vi "dfd_Get Multirate Block Params.vi"(6 "fs in [Hz]":dbl=1.0, 8 "error in (no error)":errorcluster, 9 "type (FLP)":enum16{"FLP", "FXP"}(ring), 11 "multirate filter in":T3={"mMRate_Structure"=enum."CIC", "mMRate_Mode"=0, "mMRate_Factor"=1, "mMRate_FIRParams"={"mMRate_FIR_H"=[], "mMRate_FIR_IsNyquist?"=FALSE, "mMRate_FIR_IsSymmetric?"=FALSE}, "mMRate_CICParams"={"mMRate_CIC_#Stage"=2, "mMRate_CIC_Lag"=1, "mMRate_CIC_Type"=enum."Lowpass"}, "mMRate_Order"=1, "mMRate_Version"="1.0", "mMRate_Comments"="1.0", "mMRate_RationalFactor"={"mMRate_L"=-1, "mMRate_M"=-1}, "mMRate_Fs"=0.0, "mMRate_Quantized?"=FALSE, "mMRate_QFilterGain"=1.0, "mMRate_CoefWl"=16, "mMRate_Scaling"={"mMRate_ScaleByPowerOf2?"=FALSE, "mMRate_ScaleType"=enum."Time Domain 1-Norm"}, "mMRate_InputWl"=0, "mMRate_OutputWl"=0, "mMRate_OutputMode"=enum."Nearest", "mMRate_MultMode"=enum."Truncated", "mMRate_BitPruning"=FALSE, "mMRate_GainWl"=16, "mMRate_OutputFwl"=0, "mMRate_SumIwl"=0, "mMRate_InputIwl "=16, "mMRate_SumWl"=32, "mMRate_CoefIwl"=0} {"mMRate_SumWl" min=1 max=32 step=1; "mMRate_InputIwl" min=1 max=32 step=1; "mMRate_GainWl" min=1 max=32 step=1; "mMRate_OutputWl" min=1 max=32 step=1; "mMRate_InputWl" min=1 max=32 step=1; "mMRate_CoefWl" min=1 max=32 step=1; "mMRate_Mode" items=["Default"=-1, "No Rate Change"=0, "Interpolation"=1, "Decimation"=2, "Interpolated"=3, "Rational"=4]}) -> (0 "error out":errorcluster, 1 "filter fs":dbl, 2 "factor":T1={"L"=1, "M"=1}, 3 "mode":T2 items=["Default"=-1, "No Rate Change"=0, "Interpolation"=1, "Decimation"=2, "Interpolated"=3, "Rational"=4], 4 "fs out [Hz]":dbl, 5 "order":i32, 7 "FIR":dbl[](array[numeric]))   [LabVIEW 2017, in "NI_DigFilterLicensed.lvlib"]
uses:
  <vilib>/addons/Digital Filter Design/NI_DigFilterLicensed.lvlib
  <vilib>/addons/Digital Filter Design/_Objects.llb/DFD Multirate Filter Obj.ctl
  <vilib>/addons/Digital Filter Design/_Objects.llb/DFD Multirate Mode.ctl
  <vilib>/addons/Digital Filter Design/_Objects.llb/DFD Coef Norm Type.ctl
  <vilib>/addons/Digital Filter Design/_Objects.llb/DFD Round-off Mode.ctl
  <vilib>/addons/Digital Filter Design/_Objects.llb/DFD FXP MRate Multiply Mode.ctl
  <vilib>/addons/Digital Filter Design/_Objects.llb/DFD Multirate Rational Factor.ctl
  <vilib>/addons/Digital Filter Design/_Misc.llb/dfd_Error Handlers (Single).vi
  <vilib>/addons/Digital Filter Design/NI_DigFilter_FXP.lvlib
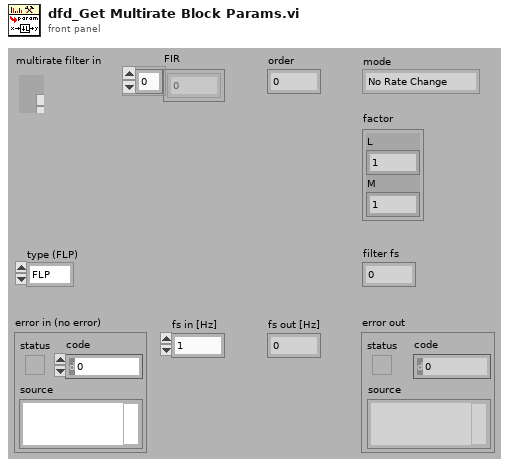
[diagram p1: front panel]
types:
  T1 = typedef "NI_DigFilterLicensed.lvlib/DFD Multirate Rational Factor.ctl" = cluster{"L":i32, "M":i32}
  T2 = typedef "NI_DigFilterLicensed.lvlib/DFD Multirate Mode.ctl" = i16
  T3 = typedef "NI_DigFilterLicensed.lvlib/DFD Multirate Filter Obj.ctl" = cluster{"mMRate_Structure":enum16{"CIC", "FIR", "IIR", "Lattice"}, "mMRate_Mode":T2, "mMRate_Factor":i32, "mMRate_FIRParams":cluster{"mMRate_FIR_H":dbl[], "mMRate_FIR_IsNyquist?":bool, "mMRate_FIR_IsSymmetric?":bool}, "mMRate_CICParams":cluster{"mMRate_CIC_#Stage":i32, "mMRate_CIC_Lag":i32, "mMRate_CIC_Type":enum16{"Lowpass", "Highpass"}}, "mMRate_Order":i32, "mMRate_Version":string, "mMRate_Comments":string, "mMRate_RationalFactor":cluster{"mMRate_L":i32, "mMRate_M":i32}, "mMRate_Fs":dbl, "mMRate_Quantized?":bool, "mMRate_QFilterGain":dbl, "mMRate_CoefWl":i16, "mMRate_Scaling":cluster{"mMRate_ScaleByPowerOf2?":bool, "mMRate_ScaleType":T4}, "mMRate_InputWl":i16, "mMRate_OutputWl":i16, "mMRate_OutputMode":T5, "mMRate_MultMode":T6, "mMRate_BitPruning":bool, "mMRate_GainWl":i16, "mMRate_OutputFwl":i16, "mMRate_SumIwl":i16, "mMRate_InputIwl ":i16, "mMRate_SumWl":i16, "mMRate_CoefIwl":i16}
  T4 = typedef "NI_DigFilterLicensed.lvlib/DFD Coef Norm Type.ctl" = enum16{"No Norm", "Time Domain 1-Norm", "Time Domain 2-Norm", "Time Domain Inf-Norm"}
  T5 = typedef "NI_DigFilterLicensed.lvlib/DFD Round-off Mode.ctl" = enum16{"Nearest", "Truncation"}
  T6 = typedef "NI_DigFilterLicensed.lvlib/DFD FXP MRate Multiply Mode.ctl" = enum16{"Truncated", "Full"}
  T7 = typedef "NI_DigFilterLicensed.lvlib/dfd_Internal Quantization Settings.ctl" = cluster{"source":T8, "wl":i16, "iwl":i16, "overflow mode":enum16{"Saturation", "Wrap"}, "rounding mode":enum16{"Nearest", "Truncation"}, "signed?":bool}
  T8 = typedef "NI_DigFilterLicensed.lvlib/dfd_Internal Quantization Srcs.ctl" = u16
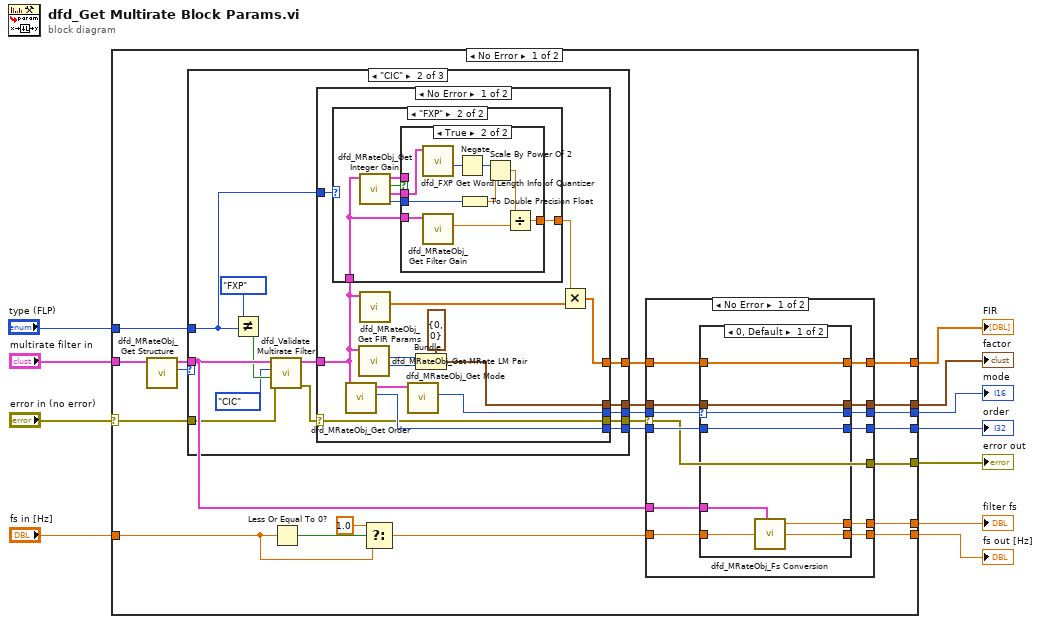
[diagram p0: block diagram]
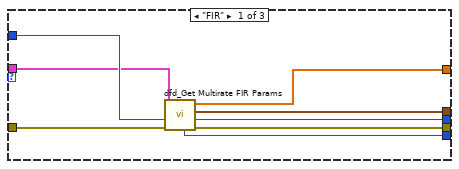
[diagram p2: hidden frame]
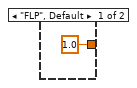
[diagram p3: hidden frame]
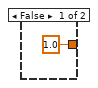
[diagram p4: hidden frame]
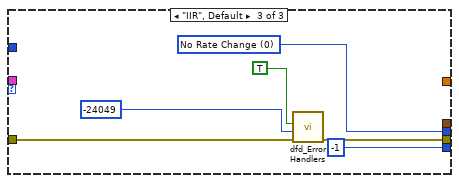
[diagram p6: hidden frame]
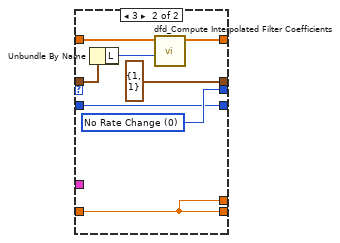
[diagram p7: hidden frame]
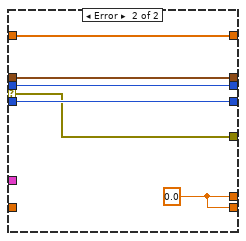
[diagram p8: hidden frame]
diagram:
  n1 = case shown="No Error" "error in (no error)" {
    selector: "error in (no error)" -> [w32 w126]
    tunnel: "multirate filter in" -> [w19 _]
    tunnel: "fs in [Hz]" -> [w29 _]
    tunnel: [w25 _] -> w8
    tunnel: [w24 _] -> w7
    tunnel: [w14 w126] -> w5
    tunnel: [w23 _] -> w6
    tunnel: "type (FLP)" -> [w20 _]
    tunnel: [w15 _] -> w3
    tunnel: [w13 _] -> w2
    tunnel: [w12 _] -> w1
    frame No Error {
      n2 = call <vilib>:"dfd_MRateObj_Get Structure.vi"("multirate filter in"=w19) -> ("structure"=w18:enum16{"CIC", "FIR", "IIR", "Lattice"}, "dup multirate filter"=w16:T3)  [unwired: 9 out]
      n3 = case shown="\"CIC\"" w18 {
        tunnel: w32 -> [w40 w43 w87]
        tunnel: [w39 w53 w88] -> w28
        tunnel: [w38 w50 _] -> w27
        tunnel: [w37 w49 w85] -> w26
        tunnel: [w36 w52 _] -> w22
        tunnel: [w35 w51 -1 ("factor")] -> w21
        tunnel: w20 -> [w34 w41 _]
        tunnel: w16 -> [w33 w47 _]
        frame "FIR" {
          n4 = call <vilib>:"dfd_Get Multirate FIR Params.vi"("error in (no error)"=w40, "type (FLP)"=w34, "multirate filter in"=w33) -> ("error out"=w39:errorcluster, "mode"=w37:T2, "factor"=w38:T1, "h (n)"=w36:dbl[], "order"=w35:i32)  [unwired: 1 in, 3 out]
        }
        frame "CIC" {
          n5 = Not Equal?(x=enum16{"FLP", "FXP"}."FXP", y=w41) -> (x != y?=w45:bool)
          n6 = call <vilib>:"dfd_Validate Multirate Filter.vi"("error in (no error)"=w43, "skip FXP? (T)"=w45, "preferred structure"=enum16{"CIC", "FIR", "IIR", "Lattice"}."CIC", "multirate filter in"=w47) -> ("error out"=w42:errorcluster, "multirate filter out"=w46:T3)  [unwired: 6 out]
          n7 = case shown="No Error" w42 {
            selector: w42 -> [w59 w84]
            tunnel: [w59 w84] -> w53
            tunnel: [w57 _] -> w52
            tunnel: [w66 _] -> w51
            tunnel: [w62 _] -> w50
            tunnel: [w60 _] -> w49
            tunnel: w46 -> [w56 _]
            tunnel: w41 -> [w54 _]
            frame No Error {
              n8 = case shown="\"FXP\"" w54 {
                tunnel: w56 -> [_ w69]
                tunnel: [1.0 w68] -> w55
                frame "FLP", Default {
                }
                frame "FXP" {
                  n9 = call <vilib>:"dfd_MRateObj_Get Integer Gain.vi"("multirate filter"=w69) -> ("I32 gain"=w71:i32, "Gain quantizer"=w72:T7, "on FPGA?"=w73:bool, "dup multirate filter"=w70:T3)  [unwired: 7 out]
                  n10 = case shown="True" w73 {
                    tunnel: w71 -> [_ w81]
                    tunnel: w72 -> [_ w79]
                    tunnel: w70 -> [_ _]
                    tunnel: w69 -> [_ w78]
                    tunnel: [1.0 w75] -> w68
                    frame False {
                    }
                    frame True {
                      n11 = call <vilib>:"dfd_FXP Get Word Length Info of Quantizer.vi"("quantization settings"=w79) -> ("fwl"=w82:i16)  [unwired: 10 out]
                      n12 = call <vilib>:"dfd_MRateObj_Get Filter Gain.vi"("multirate filter in"=w78) -> ("gain"=w76:dbl)  [unwired: 10 out]
                      n13 = Negate(x=w82) -> (-x=w83:i16)
                      n14 = To Double Precision Float(number=w81) -> (double precision float=w80:dbl)
                      n15 = Scale By Power Of 2(n=w83, x=w80) -> (x*2^n=w77:dbl)
                      n16 = Divide(x=w77, y=w76) -> (x/y=w75:dbl)
                    }
                  }
                }
              }
              n17 = call <vilib>:"dfd_MRateObj_Get Order.vi"("multirate filter in"=w56) -> ("order"=w66:i32, "dup multirate filter"=w61:T3)  [unwired: 9 out]
              n18 = call <vilib>:"dfd_MRateObj_Get MRate LM Pair.vi"("multirate filter in"=w56) -> ("M"=w64:i32, "L"=w65:i32)  [unwired: 1 in, 8 out]
              n19 = call <vilib>:"dfd_MRateObj_Get FIR Params.vi"("multirate filter in"=w56) -> ("h(n)"=w58:dbl[])  [unwired: 10 out]
              n20 = call <vilib>:"dfd_MRateObj_Get Mode.vi"("multirate filter in"=w61) -> ("mode"=w60:T2)  [unwired: 10 out]
              n21 = Bundle(cluster=T1 {"L"=0, "M"=0} ("factor"), "L"=w65, "M"=w64) -> (w62:T1)
              n22 = Multiply(x=w55, y=w58) -> (x*y=w57:dbl[])
            }
            frame Error {
            }
          }
        }
        frame "IIR", Default {
          w85 = T2 0 items=["Default"=-1, "No Rate Change"=0, "Interpolation"=1, "Decimation"=2, "Interpolated"=3, "Rational"=4] ("mode")
          n23 = call-poly <vilib>:"dfd_Error Handlers.vi"("error in (no error)"=w87, "error code"=-24049 ("ERR_INVALID_MULTIRATE_FILTER"), "condition failed?"=TRUE) -> ("error out"=w88:errorcluster)  [unwired: 8 out]
        }
      }
      n24 = Less Or Equal To 0?(x=w29) -> (x <= 0?=w31:bool)
      n25 = Select(t=1.0, s=w31, f=w29) -> (s? t:f=w17:dbl)
      n26 = case shown="No Error" w28 {
        selector: w28 -> [w91 w121]
        tunnel: w27 -> [w100 w125]
        tunnel: w26 -> [w102 w124]
        tunnel: [w99 w125] -> w25
        tunnel: [w98 w124] -> w24
        tunnel: w17 -> [w95 _]
        tunnel: [w96 w123] -> w23
        tunnel: w21 -> [w97 w123]
        tunnel: w22 -> [w103 w122]
        tunnel: w16 -> [w93 _]
        tunnel: [w101 w122] -> w15
        tunnel: [w94 w120] -> w12
        tunnel: [w92 w120] -> w13
        tunnel: [w91 w121] -> w14
        frame No Error {
          n27 = case shown="0, Default" w102 {
            selector: w102 -> [w109 _]
            tunnel: w103 -> [w111 w119]
            tunnel: [w111 w118] -> w101
            tunnel: w100 -> [w110 w117]
            tunnel: [w110 T1 {"L"=1, "M"=1} ("factor")] -> w99
            tunnel: [w109 w115] -> w98
            tunnel: [w108 w112] -> w96
            tunnel: w97 -> [w108 w112]
            tunnel: w95 -> [w107 w114]
            tunnel: [w106 w114] -> w94
            tunnel: w93 -> [w105 _]
            tunnel: [w104 w114] -> w92
            frame 0, Default {
              n28 = call <vilib>:"dfd_MRateObj_Fs Conversion.vi"("multirate filter"=w105, "fsin"=w107) -> ("filter fs"=w104:dbl, "fsout"=w106:dbl)  [unwired: 4 out]
            }
            frame 3 {
              w115 = T2 0 items=["Default"=-1, "No Rate Change"=0, "Interpolation"=1, "Decimation"=2, "Interpolated"=3, "Rational"=4] ("mode")
              n29 = Unbundle By Name(w117) -> ("L"=w113:i32)
              n30 = call <vilib>:"dfd_Compute Interpolated Filter Coefficients.vi"("factor"=w113, "numerator in"=w119) -> ("numerator out"=w118:dbl[])  [unwired: 2 in, 7 out]
            }
          }
        }
        frame Error {
          w120 = 0.0 ("fs in [Hz]")
        }
      }
    }
    frame Error {
    }
  }
  "mode" <- w7
  "factor" <- w8
  "fs out [Hz]" <- w1
  "filter fs" <- w2
  "error out" <- w5
  "order" <- w6
  "FIR" <- w3
